vi "Create Dataset DB.vi"(6 "Local Data in":T1, 8 "error in (no error)":errorcluster) -> (0 "error out":errorcluster, 4 "Local Data out":T1)   [LabVIEW 2024]
uses:
  Controls/RVHR - Local Data.ctl
  Controls/Test Cluster.ctl
  Controls/Excluded Information.ctl
  Controls/Language.ctl
  Controls/Device_Type.ctl
  <vilib>/Utility/miscctls.llb/LVRectTypeDef.ctl
  <vilib>/Utility/miscctls.llb/LVBoundsTypeDef.ctl
  <vilib>/drjdpowell/SQLite Library/SQL Connection/Open (path).vi
  <vilib>/drjdpowell/SQLite Library/SQL Connection/Open (string).vi
  <vilib>/AdvancedString/Path To Command Line String.vi
  <vilib>/drjdpowell/SQLite Library/SQL Connection/Execute SQL (No results).vi
  <vilib>/drjdpowell/SQLite Library/SQL Connection/Connection.lvclass
  <vilib>/drjdpowell/SQLite Library/SQLite.lvlib
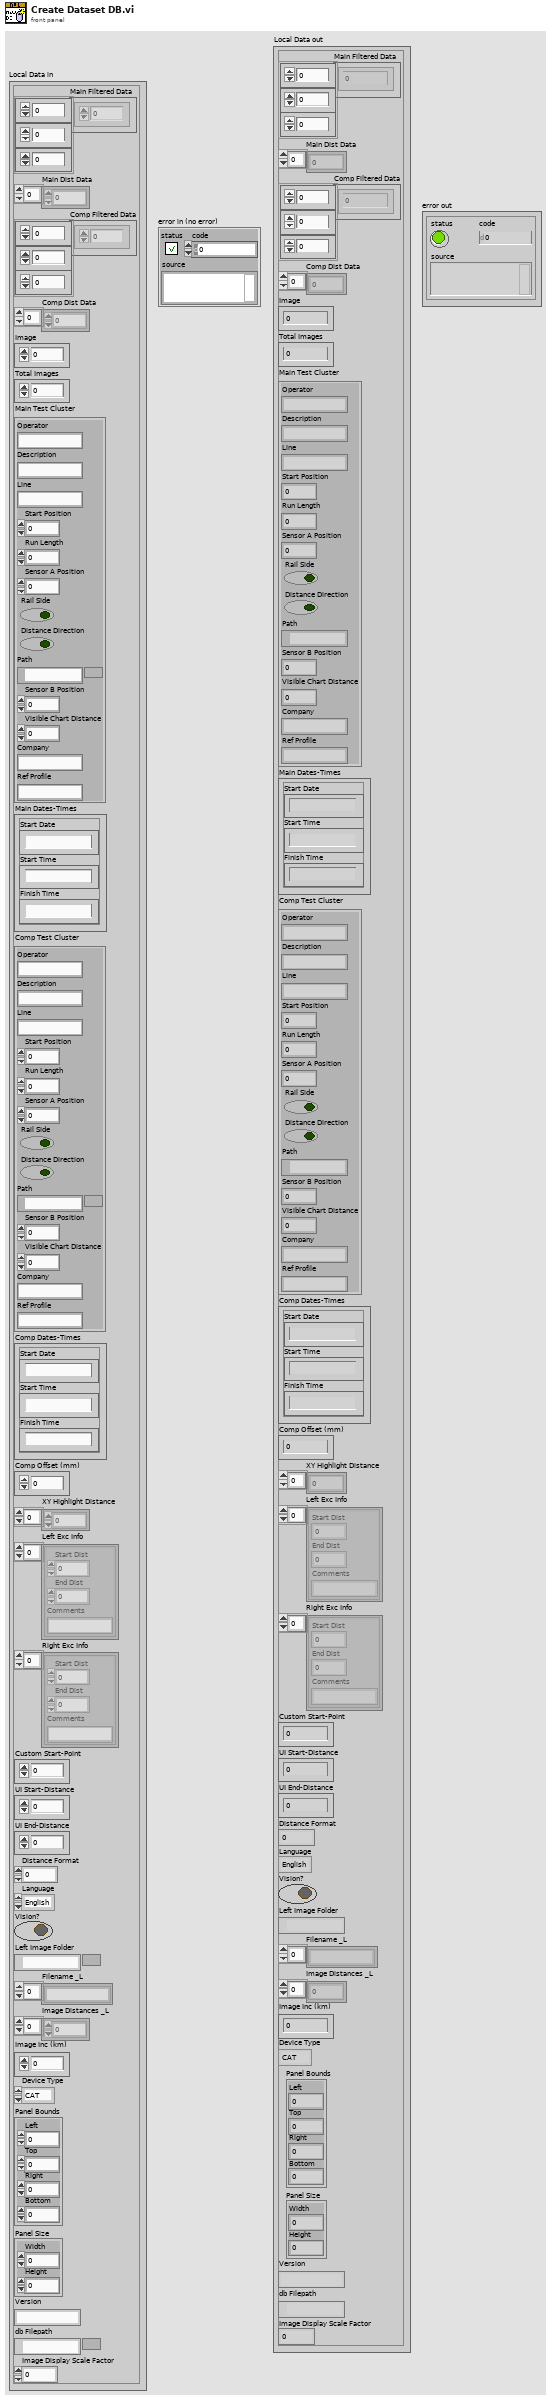
[diagram p1: front panel]
types:
  T1 = typedef "RVHR - Local Data.ctl" = cluster{"Main Filtered Data":dbl[][][], "Main Dist Data":dbl[], "Comp Filtered Data":dbl[][][], "Comp Dist Data":dbl[], "Image":u16, "Total Images":u16, "Main Test Cluster":T2, "Main Dates-Times":cluster{"Start Date":string, "Start Time":string, "Finish Time":string}, "Comp Test Cluster":T2, "Comp Dates-Times":cluster{"Start Date":string, "Start Time":string, "Finish Time":string}, "Comp Offset (mm)":i64, "XY Highlight Distance":dbl[], "Left Exc Info":T3[], "Right Exc Info":T3[], "Custom Start-Point":dbl, "UI Start-Distance":dbl, "UI End-Distance":dbl, "Distance Format":u8, "Language":T4, "Vision?":bool, "Left Image Folder":path, "Filename _L":string[], "Image Distances _L":dbl[], "Image Inc (km)":dbl, "Device Type":T5, "Panel Bounds":T6, "Panel Size":T7, "Version":string, "db Filepath":path, "Image Display Scale Factor":dbl}
  T2 = typedef "Test Cluster.ctl" = cluster{"Operator":string, "Description":string, "Line":string, "Start Position":dbl, "Run Length":dbl, "Sensor A Position":dbl, "Rail Side":bool, "Distance Direction":bool, "Path":path, "Sensor B Position":dbl, "Visible Chart Distance":dbl, "Company":string, "Ref Profile":string}
  T3 = typedef "Excluded Information.ctl" = cluster{"Start Dist":dbl, "End Dist":dbl, "Comments":string}
  T4 = typedef "Language.ctl" = enum16{"English", "Chinese", "German"}
  T5 = typedef "Device_Type.ctl" = enum16{"CAT", "Bi-CAT", "YRCA", "RCA", "RV-HR", "TV-HR"}
  T6 = typedef "LVRectTypeDef.ctl" = cluster{"Left":i16, "Top":i16, "Right":i16, "Bottom":i16}
  T7 = typedef "LVBoundsTypeDef.ctl" = cluster{"Width":u32, "Height":u32}
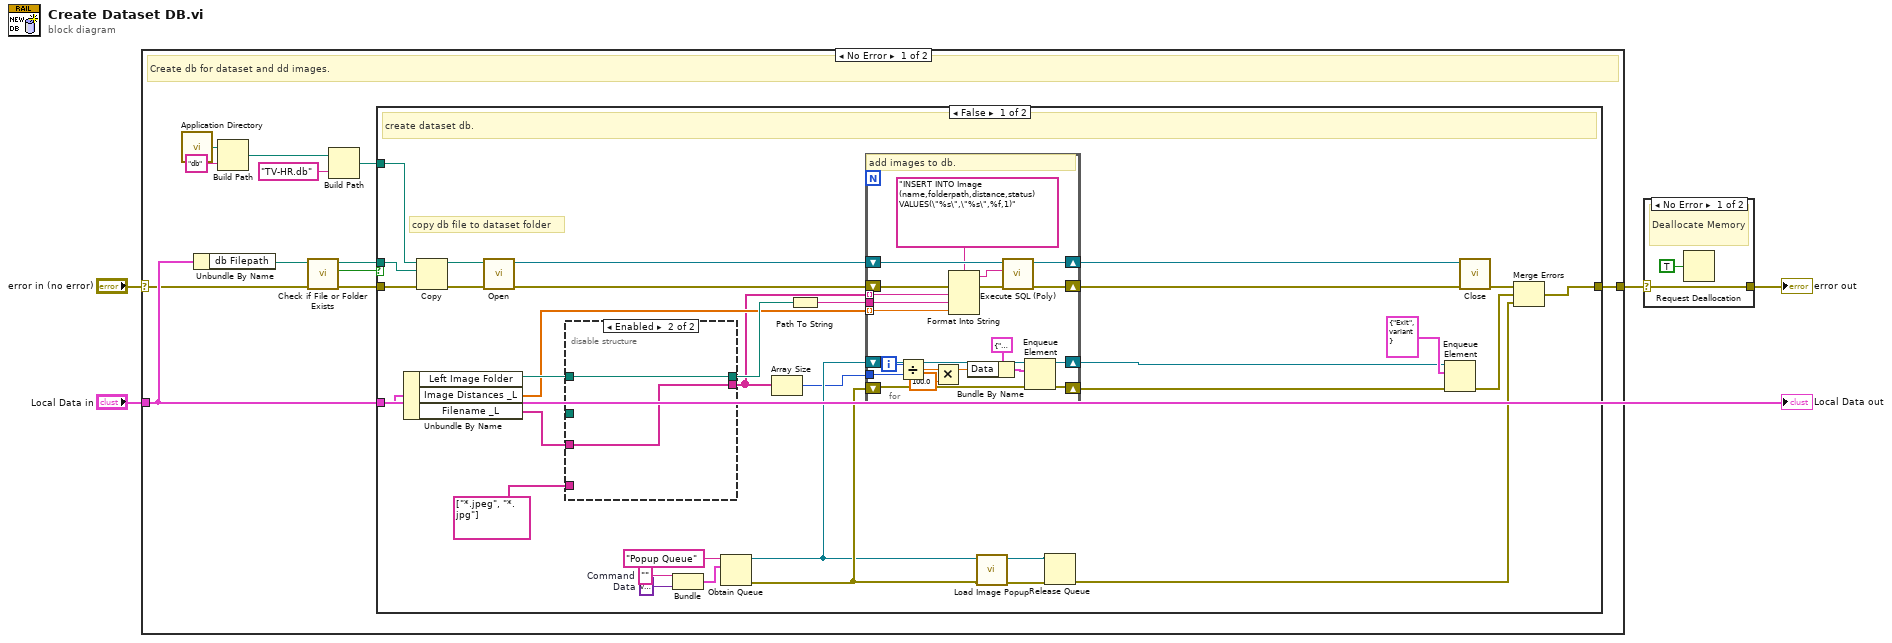
[diagram p0: block diagram]
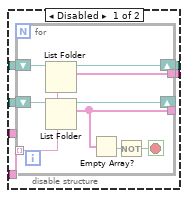
[diagram p3: hidden frame]
diagram:
  n1 = case shown="No Error" "error in (no error)" {
    selector: "error in (no error)" -> [w6 w87]
    tunnel: [w8 w87] -> w2
    tunnel: "Local Data in" -> [w7 _]
    frame No Error {
      # "Create db for dataset and dd images."
      n2 = call <vilib>:"Application Directory.vi"() -> ("Application Directory"=w15:path)
      n3 = Unbundle By Name(w7) -> ("db Filepath"=w5:path)
      n4 = Build Path(base path=w15, name or relative path="db" ("string")) -> (appended path=w13:path)
      n5 = call <vilib>:"Check if File or Folder Exists.vi"("error in (no error)"=w6, "path"=w5) -> ("error out"=w9:errorcluster, "file or folder exists?"=w16:bool, "dup path"=w10:path)  [unwired: 7 in]
      n6 = Build Path(base path=w13, name or relative path="TV-HR.db" ("string")) -> (appended path=w11:path)
      n7 = case shown="False" w16 {
        tunnel: w11 -> [w48 _]
        tunnel: w10 -> [w47 _]
        tunnel: w9 -> [w46 w86]
        tunnel: w7 -> [w43 _]
        tunnel: [w27 w86] -> w8
        frame False {
          w31 = variant  # Data
          w32 = ""  # Command
          # "copy db file to dataset folder"
          # "create dataset db."
          n8 = Unbundle By Name(w43) -> ("Left Image Folder"=w42:path, "Image Distances _L"=w37:dbl[], "Filename _L"=w22:string[])
          n9 = Copy(8:w46, 10:w47, 11:w48) -> (0:w44:errorcluster, 3:w45:path)  [unwired: 2 in, 1 out]
          n10 = call-poly <vilib>:"Open.vi"("error in (no error)"=w44, "db file"=w45) -> ("error out"=w40:errorcluster, "SQLite Connection"=w41:refnum<class "Connection.lvclass">)  [unwired: 8 in]
          n11 = disable-structure shown="Enabled" {
            disable-tunnel: w42 -> [w53 w64]
            disable-tunnel: _ -> [w52 _]
            disable-tunnel: [w51 w64] -> w39
            disable-tunnel: string[] ["*.jpeg", "*.jpg"] -> [w50 _]
            disable-tunnel: [w49 w63] -> w29
            disable-tunnel: w22 -> [_ w63]
            frame Disabled {
              n12 = for {
                tunnel: w50 -> [w60] mode=indexing
                tunnel: [w57] -> w49
                tunnel: [w56] -> _
                shift-right: [w59] -> w51
                shift-left: w53 -> [w62]
                shift-right: [w58] -> _
                shift-left: w52 -> [w61]
                stop <- w54 stop-if-true
                n13 = List Folder(path=w62, pattern=w60) -> (path out=w59:path, filenames=w57:string[])  [unwired: 2 in, 2 out]
                n14 = List Folder(path=w61, pattern=w60) -> (path out=w58:path, filenames=w56:string[])  [unwired: 2 in, 2 out]
                n15 = Empty Array?(array=w56) -> (empty?=w55:bool)
                n16 = Not(x=w55) -> (.not. x?=w54:bool)
              }
            }
            frame Enabled {
            }
          }
          n17 = Bundle("Command"=w32, "Data"=w31) -> (w34:cluster{"Command":string, "Data":variant})  [unwired: 1 in]
          n18 = Obtain Queue(name (unnamed)="Popup Queue", element data type=w34) -> (queue out=w23:refnum<queue>, error out=w28:errorcluster)  [unwired: 3 in, 1 out]
          n19 = Array Size(array=w29) -> (size(s)=w17:i32)
          n20 = Path To String(path=w39) -> (string=w38:string)
          n21 = for {
            shift-right: [w84] -> w19
            shift-left: w41 -> [w85]
            shift-right: [w83] -> w18
            shift-left: w40 -> [w82]
            tunnel: w38 -> [w78]
            tunnel: w29 -> [w77] mode=indexing
            tunnel: w37 -> [w76] mode=indexing
            tunnel: w17 -> [w72]
            shift-right: [w68] -> w20
            shift-left: w28 -> [w69]
            shift-right: [w65] -> w21
            shift-left: w23 -> [w70]
            i -> [w73]
            # "add images to db."
            n22 = Divide(x=w73, y=w72) -> (x/y=w71:dbl)
            n23 = Multiply(x=w71, y=100.0) -> (x*y=w67:dbl)
            n24 = Format Into String(format string="INSERT INTO Image (name,folderpath,distance,status) VALUES(\"%s\",\"%s\",%f,1)", error in=w82, w77, w78, w76) -> (resulting string=w80:string, error out=w81:errorcluster)  [unwired: 1 in]
            n25 = Bundle By Name(cluster=cluster{"Command":string, "Data":variant} {"Command"="Update Progress", "Data"=variant} ("output cluster"), "Data"=w67) -> (w75:cluster{"Command":string, "Data":variant})
            n26 = call-poly <vilib>:"Execute SQL (Poly).vi"("error in (no error)"=w81, "SQL"=w80, "SQLite Connection in"=w85) -> ("error out"=w83:errorcluster, "SQLite Connection"=w84:refnum<class "Connection.lvclass">)  [unwired: 7 in]
            n27 = Enqueue Element(queue=w70, element=w75, error in (no error)=w69) -> (queue out=w65:refnum<queue>, error out=w68:errorcluster)  [unwired: 1 in, 1 out]
          }
          n28 = call "Load Image Popup.vi"("error in"=w28, "queue in"=w23) -> ("error out"=w25:errorcluster)  [unwired: 8 in, 1 out]
          n29 = Release Queue(queue=w23, error in (no error)=w25) -> (error out=w24:errorcluster)  [unwired: 1 in, 2 out]
          n30 = Enqueue Element(queue=w21, element=cluster{"Command":string, "Data":variant} {"Command"="Exit", "Data"=variant} ("output cluster"), error in (no error)=w20) -> (error out=w26:errorcluster)  [unwired: 1 in, 2 out]
          n31 = call-dynamic "Close.vi"("error in (no error)"=w18, "SQLite Connection in"=w19) -> ("error out"=w36:errorcluster)  [unwired: 9 in]
          n32 = Merge Errors(w36, w26, w24) -> (w27:errorcluster)
        }
        frame True {
          # "db already exists, do nothing."
        }
      }
    }
    frame Error {
    }
  }
  n33 = case shown="No Error" w2 {
    selector: w2 -> [w88 w90]
    tunnel: [w88 w90] -> w1
    frame No Error {
      # "Deallocate Memory"
      n34 = Request Deallocation(TRUE ("flag")) -> ()
    }
    frame Error {
    }
  }
  "error out" <- w1
  "Local Data out" <- "Local Data in"
